vi "MGCC_Version2_MGCC_FntStaMach_Visualization_OpalRT_HTBtwoBatt.vi"() -> ()   [LabVIEW 2016]
uses:
  Communication/Global communication.vi
  Communication/Global communication output.vi
  Resynchronization/MGCC_Resync_global.vi
  Model Management/Global_MdlMgmt.vi
  Active and reactive power balance/MGCC_PQBal_Globals.vi
  Load Forecasting/Sub-VIs/Load_Mode.vi
  Islanded Control (He Yin)/MGCC_IsdCon_global1.vi
  PV Forecasting/Sub-VIs/f_MGCC_PVFcst_ActualPV.vi
  Energy Management (Mike)/Sub-VIs/CostSavings.vi
  Energy Management (Mike)/Sub-VIs/Battery Dispatch.vi
  Abnormal Fault State Control/Sub_VIs/Fault_Abnormal_state.vi
  Finite State Machine (He Yin)/Sub-VIs/MGCC_FntStaMach_gobal.vi
panel:
  out "Array":i32[](array[numeric])
  out "source":string
  in  "OK Button":bool
  out "l6 lockout":bool
  out "I6 fault":bool
  out "I7 lockout":bool
  out "I7 fault":bool
  out "APF 7":dbl format="%#.4f"
  out "APF 6":dbl format="%#.4f"
  out "I 7":dbl format="%#.4f"
  out "I 6":dbl format="%#.4f"
  out "L7":bool
  out "W9":bool
  out "I6":bool
  out "I7":bool
  out "L6":bool
  out "I8 fault":bool
  out "W5":bool
  out "I8 lockout":bool
  out "I2 lockout":bool
  out "I1 lockout":bool
  out "I1 Fault":bool
  out "W3":bool
  out "I4 lockout":bool
  out "I4 fault":bool
  out "I3 lockout":bool
  out "I3 fault":bool
  out "I5 lockout":bool
  out "I5 fault":bool
  out "I2 fault":bool
  out "Working state":string
  out "Red":bool
  out "Orange":bool
  out "Yellow":bool
  out "Green":bool
  out "Battery Dispatch GC":dbl[](graph)
  out "Savings":dbl
  out "Communication":bool
  out "PV Forecast":dynamicdata(graph)
  out "APF 8":dbl format="%#.4f"
  out "APF 5":dbl format="%#.4f"
  out "APF 4":dbl format="%#.4f"
  out "APF 3":dbl format="%#.4f"
  out "APF 2":dbl format="%#.4f"
  out "APF 1":dbl format="%#.4f"
  out "?":bool
  out "?":bool
  out "?":bool
  in  "Load Mode":bool
  in  "?":dbl(slide) scale=0.0..2.0
  in  "PV Mode":bool
  out "Communication":bool
  out "Active power control":bool
  out "Reactive power control":bool
  out "Output":dbl format="%#_4f"
  out "Communication":bool
  out "Resynchronization":bool
  out "Active power control":bool
  out "Reactive power control":bool
  out "SOC 3":dbl format="%#_4f"
  out "Output":dbl format="%#_4f"
  out "Communication":bool
  out "Resynchronization":bool
  out "Active power control":bool
  out "Reactive power control":bool
  out "SOC":dbl format="%#_4f"
  out "Output":dbl format="%#_4f"
  out "I 8":dbl format="%#.4f"
  out "I 5":dbl format="%#.4f"
  out "I 4":dbl format="%#.4f"
  out "I 3":dbl format="%#.4f"
  out "I 2":dbl format="%#.4f"
  out "I 1":dbl format="%#.4f"
  out "Current State":string
  out "Model Mgmt.":bool
  out "PV Forecasting":bool
  out "Load Forecasting":bool
  out "PQ Balance":bool
  out "Black Start":bool
  out "Data Logging":bool
  out "State Estimation":bool
  out "Energy Mgmt.":bool
  out "L6":cluster{dbl[], dbl[]}(graph)
  out "L7":cluster{dbl[], dbl[]}(graph)
  out "L8":cluster{dbl[], dbl[]}(graph)
  out "B10":cluster{dbl[], dbl[]}(graph)
  out "PV":cluster{dbl[], dbl[]}(graph)
  out "L11":cluster{dbl[], dbl[]}(graph)
  out "L5":cluster{dbl[], dbl[]}(graph)
  out "G4":cluster{dbl[], dbl[]}(graph)
  out "B12":cluster{dbl[], dbl[]}(graph)
  out "L3":cluster{dbl[], dbl[]}(graph)
  out "L2":cluster{dbl[], dbl[]}(graph)
  out "G1":cluster{dbl[], dbl[]}(graph)
  in  "Stop":bool
  in  "RESET":bool
  in  "G2":bool
  in  "G1":bool
  in  "Ready for STD":bool
  in  "Recon cmd":bool
  in  "BKS cmd":bool
  in  "island cmd":bool
  out "Sources Power":T1(graph)
  in  "Power Tabs":T2(tab)
  out "Loads Power 2":dbl(graph)
  out "Loads Power 3":dbl(graph)
  out "Loads Power 5":dbl(graph)
  out "Loads Power 6":dbl(graph)
  out "Loads Power 7":dbl(graph)
  out "Loads Power 8":dbl(graph)
  out "Loads Power 11":dbl(graph)
  in  "Voltage Tabs":T2(tab)
  out "Voltage 2":dbl(graph)
  out "Voltage 3":dbl(graph)
  out "Voltage 5":dbl(graph)
  out "Voltage 6":dbl(graph)
  out "Voltage 7":dbl(graph)
  out "Voltage 8":dbl(graph)
  out "Voltage 11":dbl(graph)
  out "L8":bool
  out "B1":bool
  out "Bess1 Slider":dbl(slide) scale=0.0..1.0
  out "PV":bool
  out "L11":bool
  out "W6":bool
  out "I8":bool
  out "W7":bool
  out "I5":bool
  out "I4":bool
  out "W4":bool
  out "I3":bool
  out "W8":bool
  out "I2":bool
  out "W2":bool
  out "I1":bool
  out "W1":bool
  out "L5":bool
  out "G4":bool
  out "B12":bool
  out "Bess2 Slider":dbl(slide) scale=0.0..1.0
  out "L3":bool
  out "L2":bool
  out "G1":bool
  # "Controller for Microgrid with Dynamic Boundary"
  # "Central Controller"
  # "BESS 12 Local Controller"
  # "BESS12"
  # "G4"
  # "L5"
  # "G1"
  # "L2"
  # "L3"
  # "Load profile \ncontrol"
  # "-Profile"
  # "-Manual"
  # "BESS10"
  # "L8"
  # "L6"
  # "PV9"
  # "L11"
  # "L7"
  # "PV9 Local Controller"
  # "BESS 10 Local Controller"
  # "-Profile"
  # "-Manual"
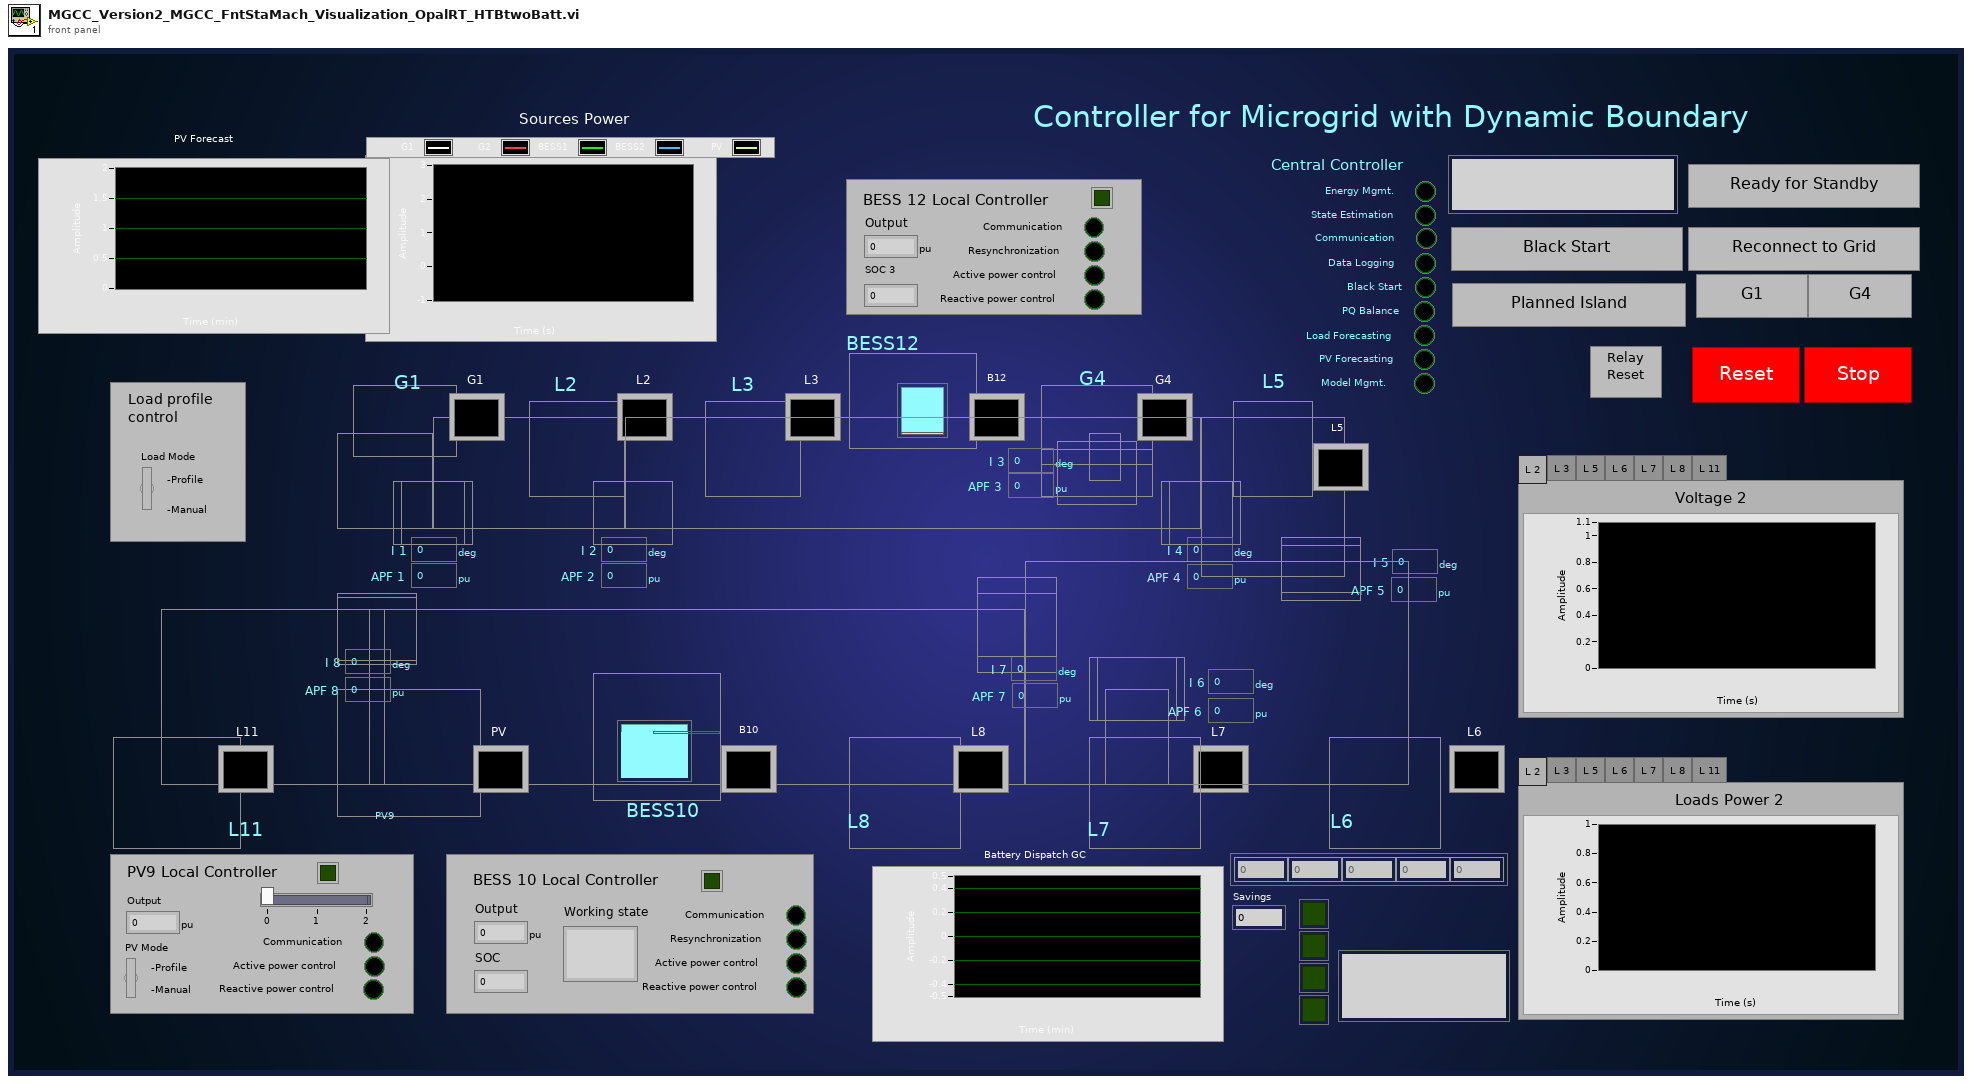
[diagram p1: front panel]
types:
  T1 = cluster{"Double":dbl, "Double":dbl, "Double":dbl, "Double":dbl, "Double":dbl}
  T2 = enum32{"L 2", "L 3", "L 5", "L 6", "L 7", "L 8", "L 11"}
  T3 = cluster{"Numeric":dbl, "Numeric":dbl, "Numeric":dbl, "Numeric":dbl}
  T4 = cluster{"Numeric":dbl, dbl, "Numeric":dbl, "Numeric":dbl, "Numeric":dbl}
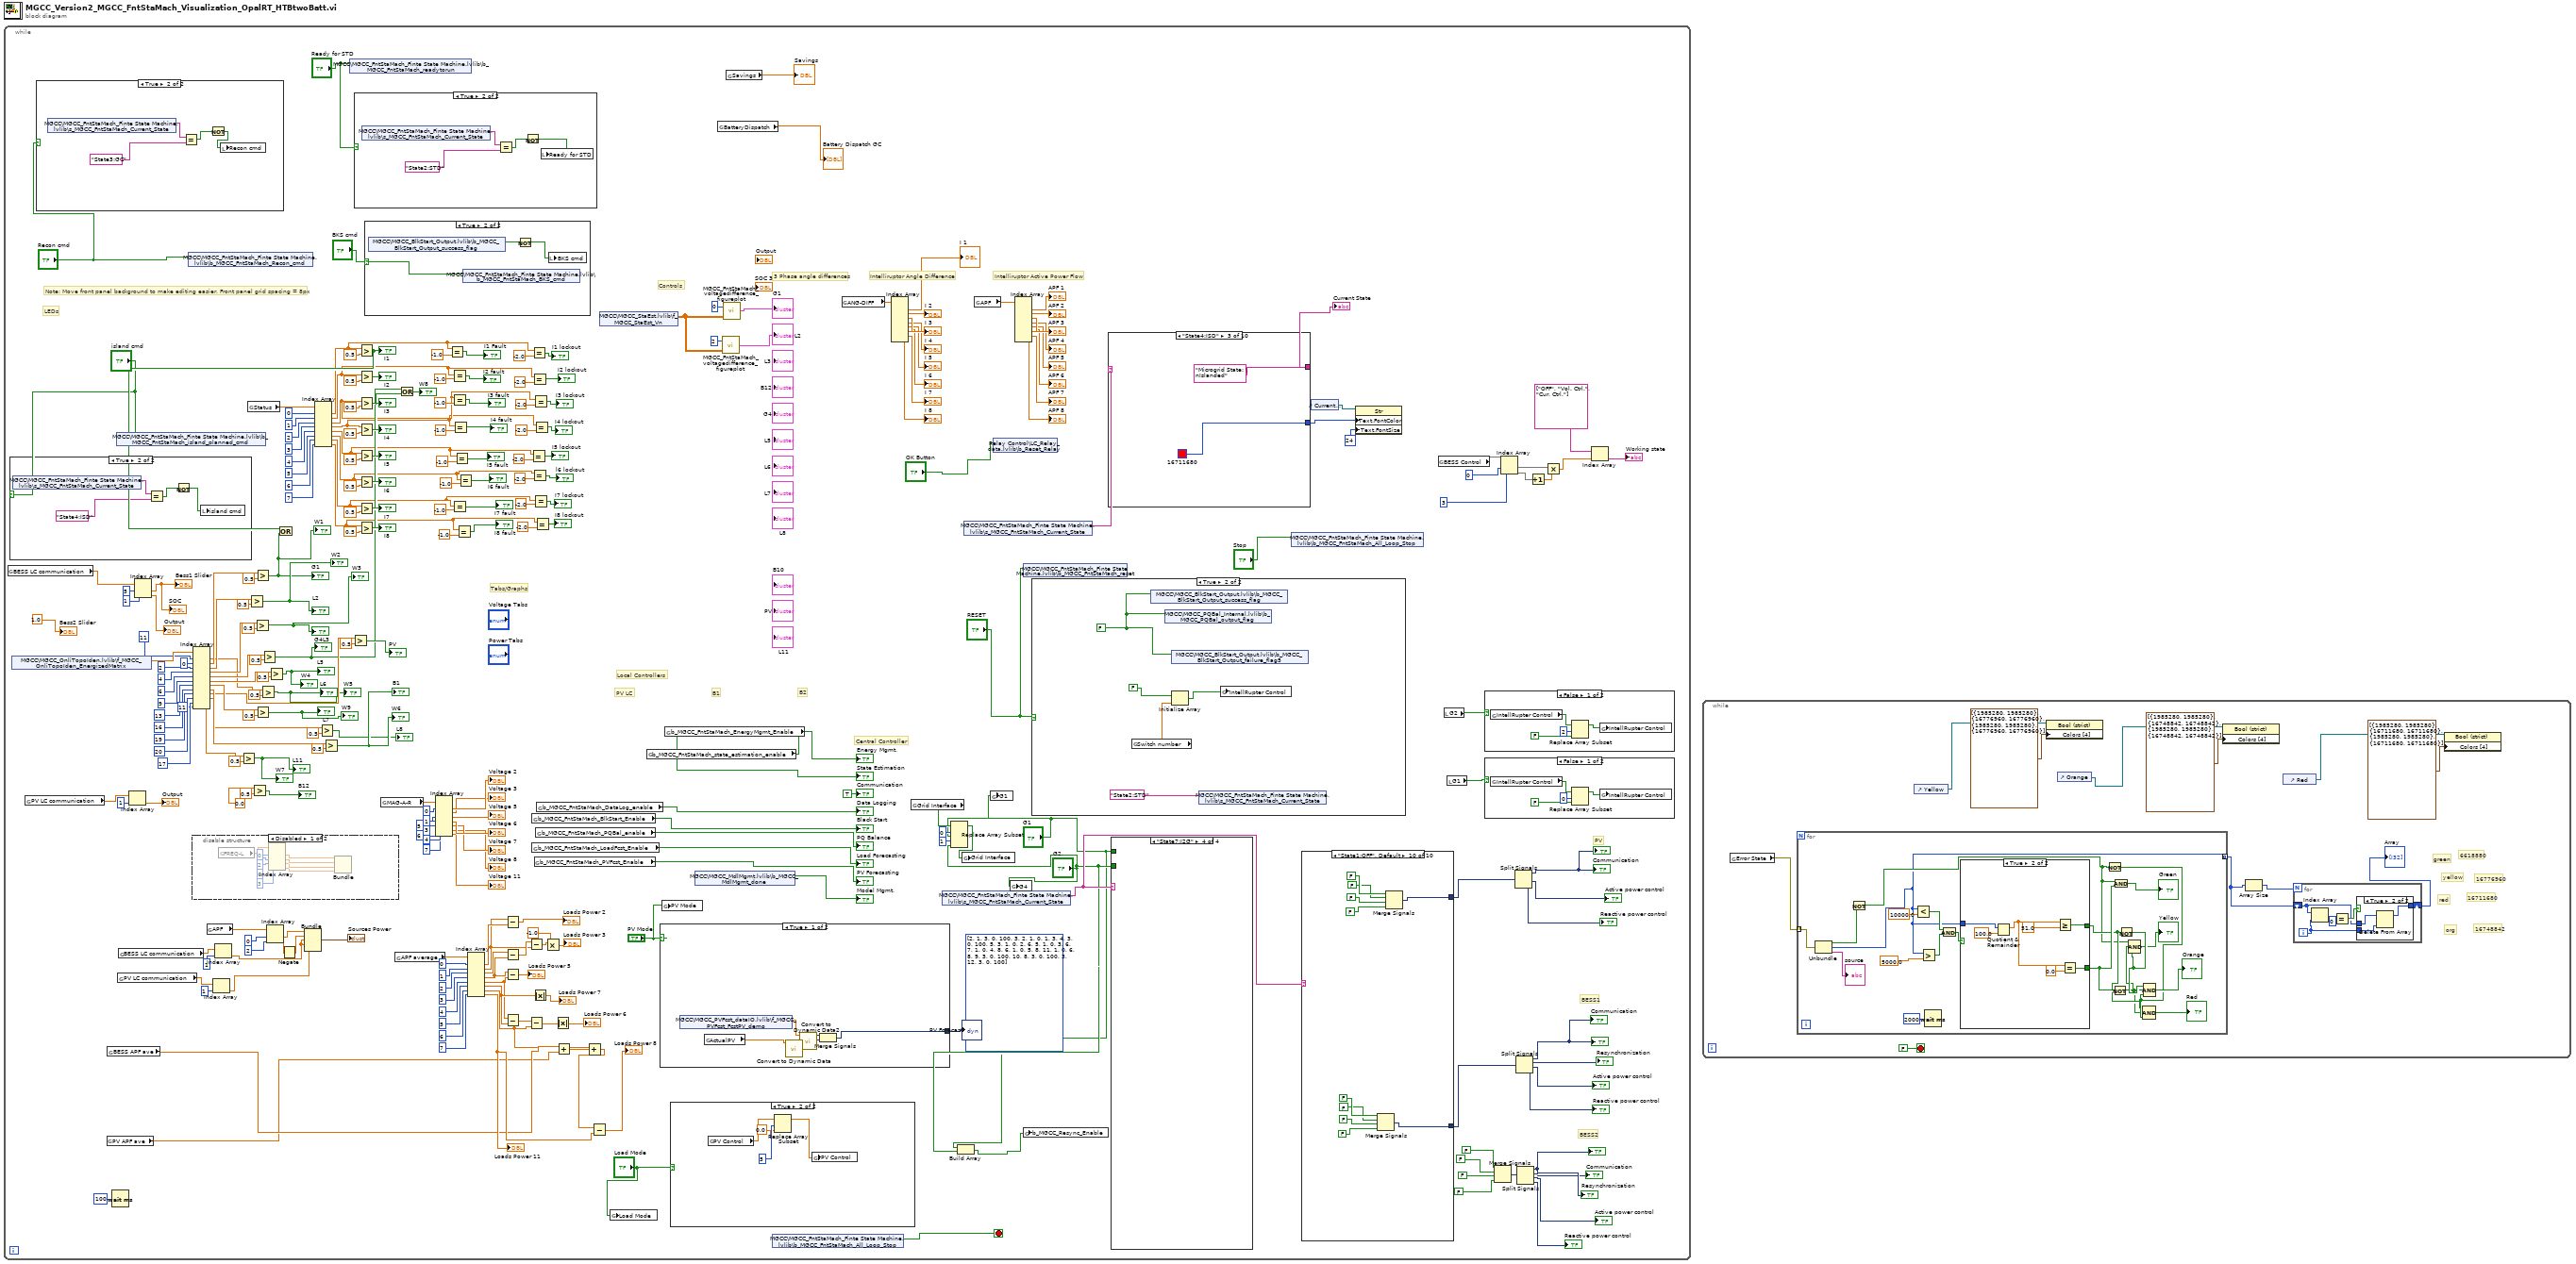
[diagram p0: block diagram]
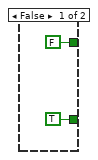
[diagram p3: hidden frame]
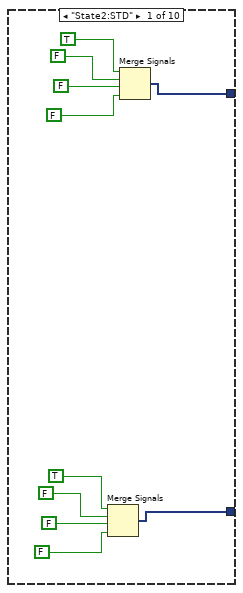
[diagram p9: hidden frame]
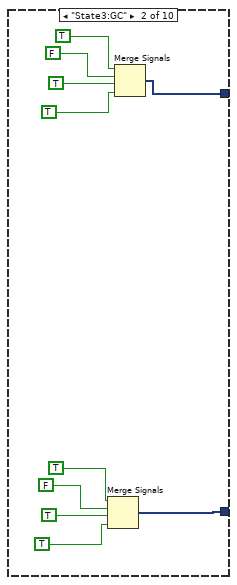
[diagram p10: hidden frame]
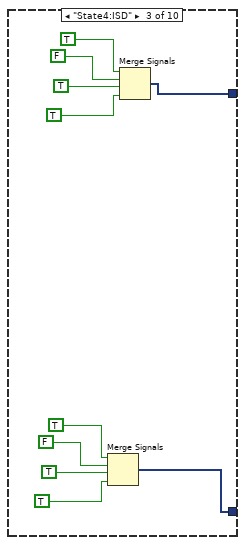
[diagram p11: hidden frame]
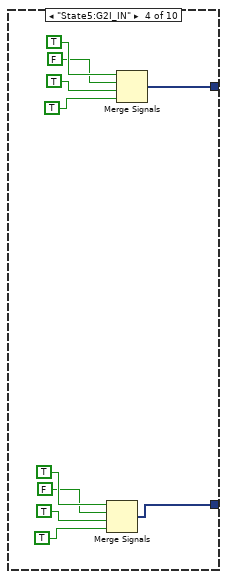
[diagram p12: hidden frame]
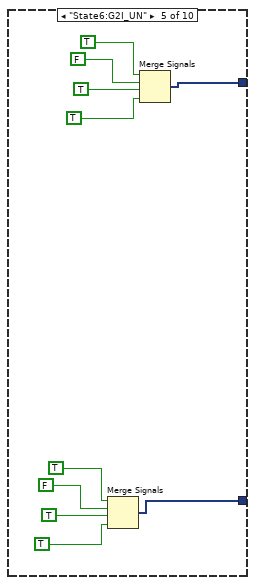
[diagram p13: hidden frame]
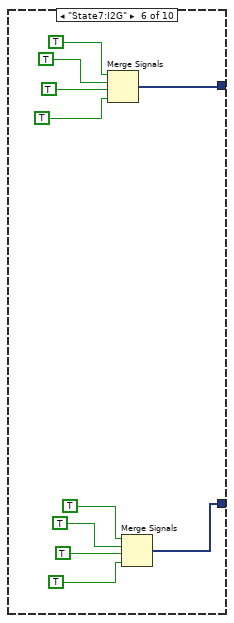
[diagram p14: hidden frame]
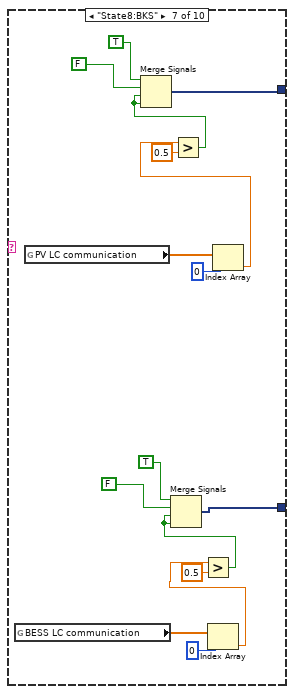
[diagram p15: hidden frame]
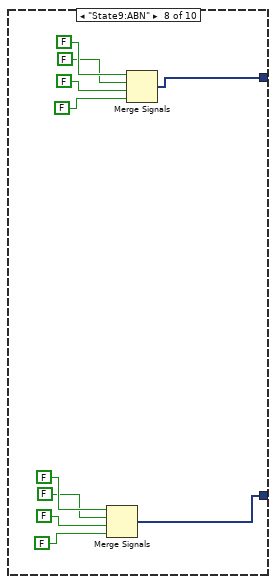
[diagram p16: hidden frame]
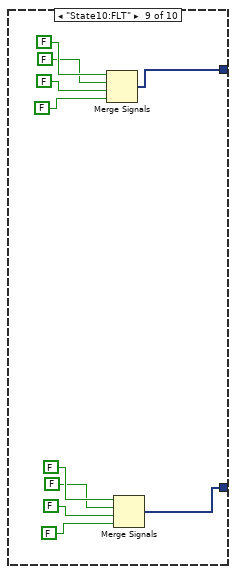
[diagram p17: hidden frame]
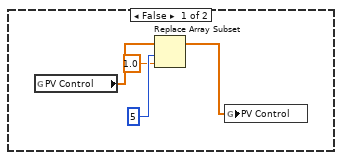
[diagram p19: hidden frame]
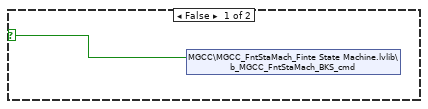
[diagram p20: hidden frame]
diagram:
  n1 = while {
    stop <- w271 stop-if-true
    (unwired) i32[][] [[2, 1, 3, 0, 100], [3, 2, 1, 0, 1], [3, 4, 3, 0, 100], [5, 3, 1, 0, 2], [6, 5, 1, 0, 3], [6, 7, 1, 0, 4], [8, 6, 1, 0, 5], [8, 11, 1, 0, 6], [8, 9, 3, 0, 100], [10, 8, 3, 0, 100], [3, 12, 3, 0, 100]]
    # "Intelliruptor Active Power Flow"
    # "BESS2"
    # "BESS1"
    # "PV"
    # "Note: Move front panel background to make editing easier. Front panel grid spacing = 8px"
    # "Intelliruptor Angle Difference"
    # "B1"
    # "Central Controller"
    # "Local Controllers"
    # "B2"
    # "PV LC"
    # "3 Phase angle differences"
    # "Controls"
    # "Tabs/Graphs"
    # "LEDs"
    n2 = global read "Global communication.vi" "BESS LC communication"() -> (w90:dbl[])
    n3 = case shown="True" "island cmd" {
      frame False {
      }
      frame True {
        n4 = shared-variable "MGCC\\MGCC_FntStaMach_Finte State Machine.lvlib\\s_MGCC_FntStaMach_Current_State"() -> (w284:string)  [unwired: 1 in, 1 out]
        n5 = Equal?(x=w284, y="State4:ISD") -> (x = y?=w282:bool)
        n6 = Not(x=w282) -> (.not. x?=w281:bool)
        n7 = local write "island cmd"(w281) -> ()
      }
    }
    n8 = shared-variable "MGCC\\MGCC_OnliTopoIden.lvlib\\f_MGCC_OnliTopoIden_EnergizedMatrix"() -> (w270:dbl[])  [unwired: 1 in, 1 out]
    n9 = global read "Global communication.vi" "PV LC communication"() -> (w84:dbl[])
    n10 = case shown="True" "Recon cmd" {
      frame False {
      }
      frame True {
        n11 = shared-variable "MGCC\\MGCC_FntStaMach_Finte State Machine.lvlib\\s_MGCC_FntStaMach_Current_State"() -> (w288:string)  [unwired: 1 in, 1 out]
        n12 = Equal?(x=w288, y="State3:GC") -> (x = y?=w286:bool)
        n13 = Not(x=w286) -> (.not. x?=w285:bool)
        n14 = local write "Recon cmd"(w285) -> ()
      }
    }
    n15 = global read "Global communication.vi" "PV APF ave"() -> (w141:dbl)
    n16 = global read "Global communication.vi" "BESS APF ave"() -> (w142:dbl)
    n17 = Wait (ms)(milliseconds to wait=u32 100) -> ()  [unwired: 1 out]
    n18 = shared-variable "MGCC\\MGCC_FntStaMach_Finte State Machine.lvlib\\b_MGCC_FntStaMach_island_planned_cmd"("island cmd") -> ()  [unwired: 1 in, 1 out]
    n19 = global read "Global communication.vi" "PV LC communication"() -> (w185:dbl[])
    n20 = global read "Global communication.vi" "BESS LC communication"() -> (w186:dbl[])
    n21 = Index Array(array=w84, index=1) -> (element=→"Output":dbl)
    n22 = Index Array(array=w90, index #1=5 ("index"), index #2=1 ("index")) -> (element #1=→"Bess1 Slider" →"SOC":dbl, element #2=→"Output":dbl)
    n23 = shared-variable "MGCC\\MGCC_FntStaMach_Finte State Machine.lvlib\\b_MGCC_FntStaMach_Recon_cmd"("Recon cmd") -> ()  [unwired: 1 in, 1 out]
    n24 = disable-structure shown="Disabled" {
      frame Disabled {
        n25 = global read "Global communication.vi" "FREQ-L"() -> (w408:dbl[])
        n26 = Index Array(array=w408, index #1=0 ("index"), index #2=2 ("index"), index #3=6 ("index"), index #4=3 ("index")) -> (element #1=w404:dbl, element #2=w403:dbl, element #3=w402:dbl, element #4=w400:dbl)
        n27 = Bundle("Numeric"=w404, "Numeric"=w403, "Numeric"=w402, "Numeric"=w400) -> (w399:T3)  [unwired: 1 in]
      }
      frame Enabled {
      }
    }
    n28 = Index Array(array=w270, index #1=11 ("index"), index #2=0 ("index"), index #3=2 ("index"), index #4=4 ("index"), index #5=6 ("index"), index #6=9 ("index"), index #7=13 ("index"), index #8=16 ("index"), index #9=19 ("index"), index #10=20 ("index"), index #11=17 ("index"), index #12=11 ("index")) -> (element #1=w241:dbl, element #2=w252:dbl, element #3=w250:dbl, element #4=w248:dbl, element #5=w245:dbl, element #6=w243:dbl, element #7=w239:dbl, element #8=w255:dbl, element #9=w234:dbl, element #10=w259:dbl, element #11=w237:dbl)  [unwired: 1 out]
    n29 = global read "Global communication.vi" "APF"() -> (w189:dbl[])
    n30 = Index Array(array=w185, index=1) -> (element=w150:dbl)
    n31 = Index Array(array=w186, index=1) -> (element=w145:dbl)
    n32 = Greater?(x=w237, y=0.5) -> (0:→"W7" →"L11":bool)
    n33 = global read "Global communication.vi" "Status"() -> (w230:dbl[])
    n34 = Greater?(x=w250, y=0.5) -> (0:→"L2" →"W2":bool)
    n35 = Greater?(x=0.0, y=0.5) -> (0:→"B12":bool)
    n36 = Greater?(x=w248, y=0.5) -> (0:→"L3" →"W3":bool)
    n37 = Greater?(x=w252, y=0.5) -> (0:w1:bool)
    "G1" <- w1
    "W1" <- w1
    n38 = Greater?(x=w239, y=0.5) -> (0:→"W9" →"L7":bool)
    n39 = Greater?(x=w241, y=0.5) -> (0:→"W5" →"L6":bool)
    n40 = Greater?(x=w245, y=0.5) -> (0:w199:bool)
    "G4" <- w199
    n41 = Index Array(array=w189, index #1=0 ("index"), index #2=2 ("index")) -> (element #1=w182:dbl, element #2=w181:dbl)
    n42 = Greater?(x=w243, y=0.5) -> (0:→"L5" →"W4":bool)
    n43 = Negate(x=w181) -> (-x=w82:dbl)
    n44 = Bundle("Numeric"=w182, w82, "Numeric"=w145, "Numeric"=w145, "Numeric"=w150) -> (→"Sources Power":T4)  [unwired: 1 in]
    n45 = Index Array(array=w230, index #1=0 ("index"), index #2=1 ("index"), index #3=2 ("index"), index #4=3 ("index"), index #5=4 ("index"), index #6=5 ("index"), index #7=6 ("index"), index #8=7 ("index")) -> (element #1=w18:dbl, element #2=w17:dbl, element #3=w16:dbl, element #4=w15:dbl, element #5=w14:dbl, element #6=w13:dbl, element #7=w12:dbl, element #8=w11:dbl)
    n46 = Greater?(x=w255, y=0.5) -> (0:→"L8":bool)
    n47 = Greater?(x=w259, y=0.5) -> (0:→"W6" →"B1":bool)
    n48 = shared-variable "MGCC\\MGCC_FntStaMach_Finte State Machine.lvlib\\b_MGCC_FntStaMach_readytorun"("Ready for STD") -> ()  [unwired: 1 in, 1 out]
    n49 = Greater?(x=w234, y=0.5) -> (0:→"PV":bool)
    n50 = case shown="True" "Ready for STD" {
      frame False {
      }
      frame True {
        n51 = shared-variable "MGCC\\MGCC_FntStaMach_Finte State Machine.lvlib\\s_MGCC_FntStaMach_Current_State"() -> (w292:string)  [unwired: 1 in, 1 out]
        n52 = Equal?(x=w292, y="State2:STD") -> (x = y?=w290:bool)
        n53 = Not(x=w290) -> (.not. x?=w289:bool)
        n54 = local write "Ready for STD"(w289) -> ()
      }
    }
    n55 = Greater?(x=w18, y=0.5) -> (0:w208:bool)
    "I1" <- w208
    n56 = Or(x=w208, y=w1) -> ()  [unwired: 1 out]
    n57 = Greater?(x=w17, y=0.5) -> (0:→"I2":bool)
    n58 = Greater?(x=w16, y=0.5) -> (0:w200:bool)
    "I3" <- w200
    n59 = Greater?(x=w15, y=0.5) -> (0:→"I4":bool)
    n60 = Greater?(x=w14, y=0.5) -> (0:→"I5":bool)
    n61 = Greater?(x=w13, y=0.5) -> (0:→"I6":bool)
    n62 = Greater?(x=w12, y=0.5) -> (0:→"I7":bool)
    n63 = Greater?(x=w11, y=0.5) -> (0:→"I8":bool)
    n64 = case shown="True" "BKS cmd" {
      selector: "BKS cmd" -> [w417 w420]
      frame False {
        n65 = shared-variable "MGCC\\MGCC_FntStaMach_Finte State Machine.lvlib\\b_MGCC_FntStaMach_BKS_cmd"(w417) -> ()  [unwired: 1 in, 1 out]
      }
      frame True {
        n66 = shared-variable "MGCC\\MGCC_BlkStart_Output.lvlib\\b_MGCC_BlkStart_Output_success_flag"() -> (w418:bool)  [unwired: 1 in, 1 out]
        n67 = shared-variable "MGCC\\MGCC_FntStaMach_Finte State Machine.lvlib\\b_MGCC_FntStaMach_BKS_cmd"(w420) -> ()  [unwired: 1 in, 1 out]
        n68 = Not(x=w418) -> (.not. x?=w419:bool)
        n69 = local write "BKS cmd"(w419) -> ()
      }
    }
    n70 = global read "Global communication.vi" "MAG-A-R"() -> (w180:dbl[])
    n71 = global read "Global communication.vi" "APF average"() -> (w165:dbl[])
    n72 = Or(x=w199, y=w200) -> (x .or. y?=→"W8":bool)
    n73 = Index Array(array=w180, index #1=0 ("index"), index #2=1 ("index"), index #3=3 ("index"), index #4=4 ("index"), index #5=5 ("index"), index #6=6 ("index"), index #7=7 ("index")) -> (element #1=→"Voltage 2":dbl, element #2=→"Voltage 3":dbl, element #3=→"Voltage 5":dbl, element #4=→"Voltage 6":dbl, element #5=→"Voltage 7":dbl, element #6=→"Voltage 8":dbl, element #7=→"Voltage 11":dbl)
    n74 = Equal?(x=w18, y=-1.0) -> (x = y?=→"I1 Fault":bool)
    n75 = Equal?(x=w17, y=-1.0) -> (x = y?=→"I2 fault":bool)
    n76 = Equal?(x=w16, y=-1.0) -> (x = y?=→"I3 fault":bool)
    n77 = Equal?(x=w12, y=-1.0) -> (x = y?=→"I7 fault":bool)
    n78 = Equal?(x=w15, y=-1.0) -> (x = y?=→"I4 fault":bool)
    n79 = Equal?(x=w14, y=-1.0) -> (x = y?=→"I5 fault":bool)
    n80 = Equal?(x=w11, y=-1.0) -> (x = y?=→"I8 fault":bool)
    n81 = Equal?(x=w13, y=-1.0) -> (x = y?=→"I6 fault":bool)
    n82 = Index Array(array=w165, index #1=0 ("index"), index #2=1 ("index"), index #3=2 ("index"), index #4=3 ("index"), index #5=4 ("index"), index #6=5 ("index"), index #7=6 ("index"), index #8=7 ("index")) -> (element #1=w156:dbl, element #2=w153:dbl, element #3=w155:dbl, element #4=w76:dbl, element #5=w75:dbl, element #6=w148:dbl, element #7=w128:dbl, element #8=w144:dbl)
    "Loads Power 11" <- w144
    n83 = Subtract(x=w153, y=w156) -> (x-y=→"Loads Power 2":dbl)
    n84 = Subtract(x=w155, y=w76) -> (x-y=w154:dbl)
    n85 = Subtract(x=w76, y=w75) -> (x-y=→"Loads Power 5":dbl)
    n86 = Subtract(x=w75, y=w148) -> (x-y=w151:dbl)
    n87 = Subtract(x=w154, y=w153) -> (x-y=w79:dbl)
    n88 = Subtract(x=w151, y=w128) -> (x-y=w147:dbl)
    n89 = Equal?(x=w14, y=-2.0) -> (x = y?=→"I5 lockout":bool)
    n90 = Equal?(x=w18, y=-2.0) -> (x = y?=→"I1 lockout":bool)
    n91 = Equal?(x=w17, y=-2.0) -> (x = y?=→"I2 lockout":bool)
    n92 = Equal?(x=w13, y=-2.0) -> (x = y?=→"l6 lockout":bool)
    n93 = global read "MGCC_FntStaMach_gobal.vi" "b_MGCC_FntStaMach_BlkStart_Enable"() -> (→"Black Start":bool)
    n94 = global read "MGCC_FntStaMach_gobal.vi" "b_MGCC_FntStaMach_LoadFcst_Enable"() -> (→"Load Forecasting":bool)
    n95 = Absolute Value(x=w148) -> (abs(x)=→"Loads Power 7":dbl)
    n96 = Equal?(x=w16, y=-2.0) -> (x = y?=→"I3 lockout":bool)
    n97 = Equal?(x=w12, y=-2.0) -> (x = y?=→"I7 lockout":bool)
    n98 = Equal?(x=w15, y=-2.0) -> (x = y?=→"I4 lockout":bool)
    n99 = Equal?(x=w11, y=-2.0) -> (x = y?=→"I8 lockout":bool)
    n100 = global read "MGCC_FntStaMach_gobal.vi" "b_MGCC_FntStaMach_PVFcst_Enable"() -> (→"PV Forecasting":bool)
    n101 = global read "MGCC_FntStaMach_gobal.vi" "b_MGCC_FntStaMach_PQBal_enable"() -> (→"PQ Balance":bool)
    n102 = global read "MGCC_FntStaMach_gobal.vi" "b_MGCC_FntStaMach_DataLog_enable"() -> (→"Data Logging":bool)
    n103 = Multiply(x=w79, y=-1.0) -> (x*y=→"Loads Power 3":dbl)
    n104 = Absolute Value(x=w147) -> (abs(x)=→"Loads Power 6":dbl)
    n105 = Add(x=w142, y=w141) -> (x+y=w129:dbl)
    n106 = Add(x=w128, y=w129) -> (x+y=w127:dbl)
    n107 = Subtract(x=w127, y=w144) -> (x-y=→"Loads Power 8":dbl)
    n108 = shared-variable "MGCC\\MGCC_StaEst.lvlib\\f_MGCC_StaEst_Vn"() -> (w62:dbl[][])  [unwired: 1 in, 1 out]
    n109 = global write "Load_Mode.vi" "Load Mode"("Load Mode") -> ()
    n110 = global read "MGCC_FntStaMach_gobal.vi" "b_MGCC_FntStaMach_state_estimation_enable"() -> (→"State Estimation":bool)
    n111 = case shown="True" "PV Mode" {
      tunnel: [w424 w427] -> w96
      frame True {
        n112 = shared-variable "MGCC\\MGCC_PVFcst_dataIO.lvlib\\f_MGCC_PVFcst_FcstPV_demo"() -> (w423:dbl[])  [unwired: 1 in, 1 out]
        n113 = global read "f_MGCC_PVFcst_ActualPV.vi" "ActualPV"() -> (w421:dbl[])
        n114 = call "Convert to Dynamic Data"("Array"=w421) -> ("Dynamic Data Type"=w425:dynamicdata)  [unwired: 3 in]
        n115 = call "Convert to Dynamic Data2"("Array"=w423) -> ("Dynamic Data Type"=w422:dynamicdata)  [unwired: 3 in]
        n116 = Merge Signals(w422, w425) -> (w424:dynamicdata)
      }
      frame False {
        n117 = global read "Global communication.vi" "PV LC communication"() -> (w429:dbl[])
        n118 = global read "Global communication output.vi" "PV Control"() -> (w433:dbl[])
        n119 = Replace Array Subset(array=w433, new element #1="?", index #1=3 ("index"), new element #2=1.0 ("new element/subarray"), index #2=4 ("index")) -> (w434:dbl[])
        n120 = Index Array(array=w429, index=1) -> (element=w426:dbl)
        n121 = global write "Global communication output.vi" "PV Control"(w434) -> ()
        n122 = Merge Signals(w426, w426) -> (w427:dynamicdata)
      }
    }
    "PV Forecast" <- w96
    n123 = global write "MGCC_PQBal_Globals.vi" "PV Mode"("PV Mode") -> ()
    n124 = global read "MGCC_FntStaMach_gobal.vi" "b_MGCC_FntStaMach_EnergyMgmt_Enable"() -> (→"Energy Mgmt.":bool)
    n125 = case shown="True" "Load Mode" {
      frame False {
        n126 = global read "Global communication output.vi" "PV Control"() -> (w411:dbl[])
        n127 = Replace Array Subset(array=w411, new element=1.0 ("new element/subarray"), index=5) -> (w412:dbl[])
        n128 = global write "Global communication output.vi" "PV Control"(w412) -> ()
      }
      frame True {
        n129 = global read "Global communication output.vi" "PV Control"() -> (w415:dbl[])
        n130 = Replace Array Subset(array=w415, new element=0.0 ("new element/subarray"), index=5) -> (w416:dbl[])
        n131 = global write "Global communication output.vi" "PV Control"(w416) -> ()
      }
    }
    n132 = shared-variable "MGCC\\MGCC_MdlMgmt.lvlib\\b_MGCC_MdlMgmt_done"() -> (→"Model Mgmt.":bool)  [unwired: 1 in, 1 out]
    n133 = global read "Battery Dispatch.vi" "BatteryDispatch"() -> (→"Battery Dispatch GC":dbl[])
    n134 = call "MGCC_FntStaMach_voltagedifference_figureplot.vi"("array"=w62, "index (row)"=2) -> ("output cluster"=→"L2":cluster{dbl[], dbl[]})
    n135 = call "MGCC_FntStaMach_voltagedifference_figureplot.vi"("array"=w62, "index (row)"=0) -> ("output cluster"=→"G1":cluster{dbl[], dbl[]})
    n136 = global read "CostSavings.vi" "Savings"() -> (→"Savings":dbl)
    n137 = shared-variable "MGCC\\MGCC_FntStaMach_Finte State Machine.lvlib\\b_MGCC_FntStaMach_All_Loop_Stop"() -> (w271:bool)  [unwired: 1 in, 1 out]
    n138 = global read "Global communication.vi" "ANG-DIFF"() -> (w140:dbl[])
    n139 = Index Array(array=w140) -> (element #1=→"I 1":dbl, element #2=→"I 2":dbl, element #3=→"I 3":dbl, element #4=→"I 4":dbl, element #5=→"I 5":dbl, element #6=→"I 6":dbl, element #7=→"I 7":dbl, element #8=→"I 8":dbl)  [unwired: 8 in]
    n140 = global read "MGCC_IsdCon_global1.vi" "Grid Interface"() -> (w72:bool[])
    n141 = shared-variable "MGCC\\MGCC_FntStaMach_Finte State Machine.lvlib\\s_MGCC_FntStaMach_Current_State"() -> (w120:string)  [unwired: 1 in, 1 out]
    n142 = Replace Array Subset(array=w72, new element #1="G1", index #1=0 ("index"), new element #2="G2", index #2=1 ("index")) -> (w71:bool[])
    n143 = Build Array("G1", "G2") -> (w131:bool[])
    n144 = global write "MGCC_IsdCon_global1.vi" "Grid Interface"(w71) -> ()
    n145 = shared-variable "MGCC\\MGCC_FntStaMach_Finte State Machine.lvlib\\s_MGCC_FntStaMach_Current_State"() -> (w197:string)  [unwired: 1 in, 1 out]
    n146 = global read "Global communication.vi" "APF"() -> (w105:dbl[])
    n147 = global write "MGCC_IsdCon_global1.vi" "G1"("G1") -> ()
    n148 = shared-variable "Relay Control\\LC_Relay_data.lvlib\\b_Reset_Relay"("OK Button") -> ()  [unwired: 1 in, 1 out]
    n149 = global write "MGCC_IsdCon_global1.vi" "G4"("G2") -> ()
    n150 = Index Array(array=w105) -> (element #1=→"APF 1":dbl, element #2=→"APF 2":dbl, element #3=→"APF 3":dbl, element #4=→"APF 4":dbl, element #5=→"APF 5":dbl, element #6=→"APF 6":dbl, element #7=→"APF 7":dbl, element #8=→"APF 8":dbl)  [unwired: 8 in]
    n151 = shared-variable "MGCC\\MGCC_FntStaMach_Finte State Machine.lvlib\\b_MGCC_FntStaMach_reset"("RESET") -> ()  [unwired: 1 in, 1 out]
    n152 = global write "MGCC_Resync_global.vi" "b_MGCC_Resync_Enable"(w131) -> ()
    n153 = case shown="True" "RESET" {
      frame False {
      }
      frame True {
        w439 = FALSE ("S0102-status-ctrl")
        n154 = global read "Global_MdlMgmt.vi" "Switch number"() -> (w436:dbl)
        n155 = shared-variable "MGCC\\MGCC_BlkStart_Output.lvlib\\b_MGCC_BlkStart_Output_success_flag"(w439) -> ()  [unwired: 1 in, 1 out]
        n156 = shared-variable "MGCC\\MGCC_PQBal_Internal.lvlib\\b_MGCC_PQBal_output_flag"(w439) -> ()  [unwired: 1 in, 1 out]
        n157 = shared-variable "MGCC\\MGCC_BlkStart_Output.lvlib\\b_MGCC_BlkStart_Output_failure_flag5"(w439) -> ()  [unwired: 1 in, 1 out]
        n158 = Initialize Array(FALSE, w436) -> (w437:bool[])
        n159 = shared-variable "MGCC\\MGCC_FntStaMach_Finte State Machine.lvlib\\s_MGCC_FntStaMach_Current_State"("State2:STD" ("s_MGCC_FntStaMach_Current_State")) -> ()  [unwired: 1 in, 1 out]
        n160 = global write "Global communication output.vi" "IntellRupter Control"(w437) -> ()
      }
    }
    n161 = case shown="\"State4:ISD\"" w197 {
      tunnel: ["Microgrid State: \nOutage" "Microgrid State: \nGrid Connected" "Microgrid State: \nIslanded" "Microgrid State: \nGrid Connected" "Microgrid State: \nGrid Connected" "Microgrid State: \nIslanded" "Microgrid State: \nIslanded" "Current State:\nAbnormal" "Current State:\nFault" "Microgrid State: \nOutage"] -> w195
      tunnel: [u32 16748842 u32 1985280 u32 16711680 u32 1985280 u32 1985280 u32 16711680 u32 16711680 u32 0 u32 0 u32 16748842] -> w194
      frame "State2:STD" {
      }
      frame "State3:GC" {
      }
      frame "State4:ISD" {
      }
      frame "State5:G2I_IN" {
      }
      frame "State6:G2I_UN" {
      }
      frame "State7:I2G" {
      }
      frame "State8:BKS" {
      }
      frame "State9:ABN" {
      }
      frame "State10:FLT" {
      }
      frame "State1:OFF", Default {
      }
    }
    "Current State" <- w195
    n162 = case shown="\"State7:I2G\"" w120 {
      tunnel: "G1" -> [_ _ _ _]
      tunnel: "G2" -> [_ _ _ _]
      frame "State6:G2I_UN" {
      }
      frame "State3:GC" {
        n163 = shared-variable "MGCC\\MGCC_Resync.lvlib\\b_MGCC_Resync_Enable"(bool[] [FALSE, FALSE] ("b_MGCC_Resync_Enable")) -> ()  [unwired: 1 in, 1 out]
      }
      frame "False", Default {
      }
      frame "State7:I2G" {
      }
    }
    n164 = shared-variable "MGCC\\MGCC_FntStaMach_Finte State Machine.lvlib\\b_MGCC_FntStaMach_All_Loop_Stop"("Stop") -> ()  [unwired: 1 in, 1 out]
    n165 = case shown="\"State1:OFF\", Default" w120 {
      tunnel: [w298 w308 w318 w328 w338 w351 w367 w374 w384 w394] -> w119
      tunnel: [w293 w304 w314 w323 w333 w343 w359 w369 w379 w389] -> w115
      frame "State2:STD" {
        n166 = Merge Signals(TRUE ("Resynchronization"), FALSE ("Resynchronization"), FALSE ("Resynchronization"), FALSE ("Resynchronization")) -> (w293:dynamicdata)
        n167 = Merge Signals(TRUE ("Resynchronization"), FALSE ("Resynchronization"), FALSE ("Resynchronization"), FALSE ("Resynchronization")) -> (w298:dynamicdata)
      }
      frame "State3:GC" {
        n168 = Merge Signals(TRUE ("Resynchronization"), FALSE ("Resynchronization"), TRUE ("Resynchronization"), TRUE ("Resynchronization")) -> (w304:dynamicdata)
        n169 = Merge Signals(TRUE ("Resynchronization"), FALSE ("Resynchronization"), TRUE ("Resynchronization"), TRUE ("Resynchronization")) -> (w308:dynamicdata)
      }
      frame "State4:ISD" {
        n170 = Merge Signals(TRUE ("Resynchronization"), FALSE ("Resynchronization"), TRUE ("Resynchronization"), TRUE ("Resynchronization")) -> (w314:dynamicdata)
        n171 = Merge Signals(TRUE ("Resynchronization"), FALSE ("Resynchronization"), TRUE ("Resynchronization"), TRUE ("Resynchronization")) -> (w318:dynamicdata)
      }
      frame "State5:G2I_IN" {
        n172 = Merge Signals(TRUE ("Resynchronization"), FALSE ("Resynchronization"), TRUE ("Resynchronization"), TRUE ("Resynchronization")) -> (w323:dynamicdata)
        n173 = Merge Signals(TRUE ("Resynchronization"), FALSE ("Resynchronization"), TRUE ("Resynchronization"), TRUE ("Resynchronization")) -> (w328:dynamicdata)
      }
      frame "State6:G2I_UN" {
        n174 = Merge Signals(TRUE ("Resynchronization"), FALSE ("Resynchronization"), TRUE ("Resynchronization"), TRUE ("Resynchronization")) -> (w333:dynamicdata)
        n175 = Merge Signals(TRUE ("Resynchronization"), FALSE ("Resynchronization"), TRUE ("Resynchronization"), TRUE ("Resynchronization")) -> (w338:dynamicdata)
      }
      frame "State7:I2G" {
        n176 = Merge Signals(TRUE ("Resynchronization"), TRUE ("Resynchronization"), TRUE ("Resynchronization"), TRUE ("Resynchronization")) -> (w351:dynamicdata)
        n177 = Merge Signals(TRUE ("Resynchronization"), TRUE ("Resynchronization"), TRUE ("Resynchronization"), TRUE ("Resynchronization")) -> (w343:dynamicdata)
      }
      frame "State8:BKS" {
        n178 = global read "Global communication.vi" "BESS LC communication"() -> (w354:dbl[])
        n179 = global read "Global communication.vi" "PV LC communication"() -> (w358:dbl[])
        n180 = Index Array(array=w354, index=0) -> (element=w353:dbl)
        n181 = Greater?(x=w353, y=0.5) -> (0:w361:bool)
        n182 = Merge Signals(TRUE ("Resynchronization"), FALSE ("Resynchronization"), w361, w361) -> (w359:dynamicdata)
        n183 = Index Array(array=w358, index=0) -> (element=w356:dbl)
        n184 = Greater?(x=w356, y=0.5) -> (0:w365:bool)
        n185 = Merge Signals(TRUE ("Resynchronization"), FALSE ("Resynchronization"), w365, w365) -> (w367:dynamicdata)
      }
      frame "State9:ABN" {
        n186 = Merge Signals(FALSE ("Resynchronization"), FALSE ("Resynchronization"), FALSE ("Resynchronization"), FALSE ("Resynchronization")) -> (w369:dynamicdata)
        n187 = Merge Signals(FALSE ("Resynchronization"), FALSE ("Resynchronization"), FALSE ("Resynchronization"), FALSE ("Resynchronization")) -> (w374:dynamicdata)
      }
      frame "State10:FLT" {
        n188 = Merge Signals(FALSE ("Resynchronization"), FALSE ("Resynchronization"), FALSE ("Resynchronization"), FALSE ("Resynchronization")) -> (w384:dynamicdata)
        n189 = Merge Signals(FALSE ("Resynchronization"), FALSE ("Resynchronization"), FALSE ("Resynchronization"), FALSE ("Resynchronization")) -> (w379:dynamicdata)
      }
      frame "State1:OFF", Default {
        n190 = Merge Signals(FALSE ("Resynchronization"), FALSE ("Resynchronization"), FALSE ("Resynchronization"), FALSE ("Resynchronization")) -> (w389:dynamicdata)
        n191 = Merge Signals(FALSE ("Resynchronization"), FALSE ("Resynchronization"), FALSE ("Resynchronization"), FALSE ("Resynchronization")) -> (w394:dynamicdata)
      }
    }
    n192 = control-ref of="Current State"() -> (w196:refnum<vi>)
    n193 = property on="Property Node" class="Str"(reference=w196, "Text.FontColor"=w194, "Text.FontSize"=u32 24 ("Text.Font:Size")) -> ()  [unwired: 1 in, 2 out]
    n194 = global read "Global communication output.vi" "BESS Control"() -> (w58)
    n195 = local read "G2"() -> (w73:bool)
    n196 = local read "G1"() -> (w74:bool)
    n197 = case shown="False" w73 {
      frame False {
        n198 = global read "Global communication output.vi" "IntellRupter Control"() -> (w276:bool[])
        n199 = Replace Array Subset(array=w276, new element=FALSE ("new element/subarray"), index=2) -> (w275:bool[])
        n200 = global write "Global communication output.vi" "IntellRupter Control"(w275) -> ()
      }
      frame True {
      }
    }
    n201 = case shown="False" w74 {
      frame False {
        n202 = global read "Global communication output.vi" "IntellRupter Control"() -> (w280:bool[])
        n203 = Replace Array Subset(array=w280, new element=FALSE ("new element/subarray"), index=0) -> (w279:bool[])
        n204 = global write "Global communication output.vi" "IntellRupter Control"(w279) -> ()
      }
      frame True {
      }
    }
    n205 = Merge Signals(FALSE ("Resynchronization"), FALSE ("Resynchronization"), FALSE ("Resynchronization"), FALSE ("Resynchronization")) -> (w106:dynamicdata)
    n206 = Index Array(array=w58, index #1=0 ("index"), index #2=3 ("index")) -> (element #1=w54, element #2=w55)
    n207 = Split Signals(w119) -> (→"Communication" →"?":dynamicdata, →"Active power control":dynamicdata, →"Reactive power control":dynamicdata)  [unwired: 4 in, 1 out]
    n208 = Split Signals(w115) -> (→"?" →"Communication":dynamicdata, →"Resynchronization":dynamicdata, →"Active power control":dynamicdata, →"Reactive power control":dynamicdata)  [unwired: 4 in]
    n209 = Split Signals(w106) -> (→"Communication" →"?":dynamicdata, →"Resynchronization":dynamicdata, →"Active power control":dynamicdata, →"Reactive power control":dynamicdata)  [unwired: 4 in]
    n210 = Increment(x=w55) -> (x+1=w53:dbl)
    n211 = Multiply(x=w54, y=w53) -> (x*y=w52:dbl)
    n212 = Index Array(array=string[] ["OFF", "Vol. Ctrl.", "Cur. Ctrl."], index=w52) -> (element=→"Working state":string)
    "Bess2 Slider" <- 1.0 ("Slide 2")
    "Communication" <- TRUE ("Communication")
  }
  n213 = while {
    stop <- FALSE stop-if-true
    # "org"
    # "16748842"
    # "red"
    # "yellow"
    # "green"
    # "16776960"
    # "16711680"
    # "6618880"
    n214 = global read "Fault_Abnormal_state.vi" "Error State"() -> (w471:errorcluster[])
    n215 = for {
      tunnel: w471 -> [w501] mode=indexing
      tunnel: [w483] -> w463 mode=indexing
      n216 = Unbundle(w501) -> ("status"=w489:bool, "code"=w483:i32, "source"=→"source":string)
      n217 = Not(x=w489) -> (.not. x?=w487:bool)
      n218 = Less?(x=w483, y=10000.0) -> (x < y?=w498:bool)
      n219 = Greater?(x=w483, y=5000.0) -> (0:w497:bool)
      n220 = Wait (ms)(milliseconds to wait=u32 2000) -> ()  [unwired: 1 out]
      n221 = And(x=w498, y=w497) -> (x .and. y?=w496:bool)
      n222 = case shown="True" w496 {
        tunnel: [FALSE w509] -> w491
        tunnel: [TRUE w506] -> w494
        tunnel: w483 -> [_ w505]
        frame False {
        }
        frame True {
          n223 = Quotient & Remainder(x=w505, y=100.0) -> (x-y*floor(x/y)=w508:dbl)  [unwired: 1 out]
          n224 = Greater Or Equal?(x=w508, y=51.0) -> (x >= y?=w509:bool)
          n225 = Equal?(x=w508, y=0.0) -> (x = y?=w506:bool)
        }
      }
      n226 = Not(x=w487) -> (.not. x?=w492:bool)
      n227 = Not(x=w494) -> (.not. x?=w486:bool)
      n228 = And(x=w487, y=w494) -> (x .and. y?=→"Green":bool)
      n229 = Not(x=w491) -> (.not. x?=w488:bool)
      n230 = Compound Arithmetic op=AND(w487, w486, w488) -> (→"Yellow":bool)
      n231 = Compound Arithmetic op=AND(w491, w486, w492) -> (→"Red":bool)
      n232 = Compound Arithmetic op=AND(w488, w486, w492) -> (→"Orange":bool)
    }
    n233 = control-ref of="Yellow"() -> (w470:refnum<vi>)
    n234 = property on="Property Node" class="Bool (strict)"(reference=w470, "Colors [4]"=cluster{u32, u32}[] [{1985280, 1985280}, {16776960, 16776960}, {1985280, 1985280}, {16776960, 16776960}]) -> ()  [unwired: 1 in, 2 out]
    n235 = control-ref of="Orange"() -> (w465:refnum<vi>)
    n236 = property on="Property Node" class="Bool (strict)"(reference=w465, "Colors [4]"=cluster{u32, u32}[] [{1985280, 1985280}, {16748842, 16748842}, {1985280, 1985280}, {16748842, 16748842}]) -> ()  [unwired: 1 in, 2 out]
    n237 = Array Size(array=w463) -> (size(s)=w462:i32)
    n238 = control-ref of="Red"() -> (w466:refnum<vi>)
    n239 = for {
      N: w462 -> [_]
      shift-right: [w474] -> w464
      shift-left: w463 -> [w473]
      i -> [w475]
      n240 = Index Array(array=w473, index=w475) -> (element=w478:i32)
      n241 = Equal?(x=w478, y=0) -> (x = y?=w476:bool)
      n242 = case shown="True" w476 {
        tunnel: w473 -> [w479 w482]
        tunnel: w475 -> [_ w481]
        tunnel: [w479 w480] -> w474
        frame False {
        }
        frame True {
          n243 = Delete From Array(array=w482, index=w481) -> (array with subset deleted=w480:i32[])  [unwired: 1 in, 1 out]
        }
      }
    }
    "Array" <- w464
    n244 = property on="Property Node" class="Bool (strict)"(reference=w466, "Colors [4]"=cluster{u32, u32}[] [{1985280, 1985280}, {16711680, 16711680}, {1985280, 1985280}, {16711680, 16711680}]) -> ()  [unwired: 1 in, 2 out]
  }
